vi "Set Column Default Width.vi"(8 "error in":errorcluster, 10 "Default Width":i32, 11 "SourceGrid in":refnum<class "SourceGrid.lvclass">) -> (0 "error out":errorcluster, 3 "SourceGrid out":refnum<class "SourceGrid.lvclass">)   [LabVIEW 2024, in "SourceGrid.lvlib" / "SourceGrid.lvclass"]
doc: "Indicates the default width of new column"
uses:
  SourceGrid.lvclass
  SourceGrid.lvclass/SourceGrid.ctl
  D:/git/Sourcegrid-LabVIEW/dll/SourceGrid.dll
  dll/SourceGrid.dll
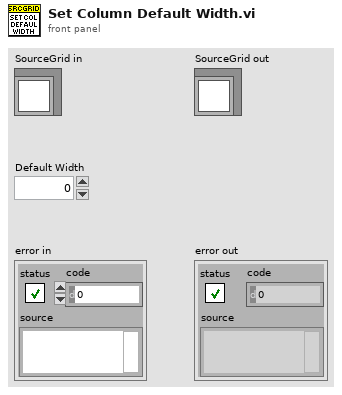
[diagram p1: front panel]
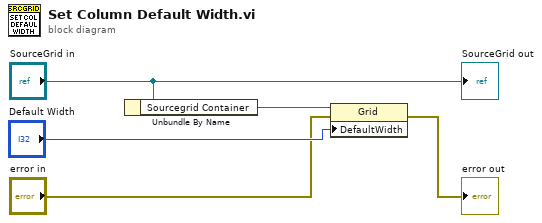
[diagram p0: block diagram]
diagram:
  n1 = Unbundle By Name("SourceGrid in") -> ("Sourcegrid Container"=w4:refnum<k24>)
  n2 = property class="Grid"(reference=w4, error in="error in", "DefaultWidth"="Default Width") -> (error out=→"error out":errorcluster)  [unwired: 1 out]
  "SourceGrid out" <- "SourceGrid in"
